vi "EncoderLimitsTurret.vi"(8 "Encoder Minimum Position":dbl, 9 "Encoder Maximum Position":dbl, 10 "Encoder Position":dbl, 11 "Output":dbl) -> (3 "Output":dbl)   [LabVIEW 2020]
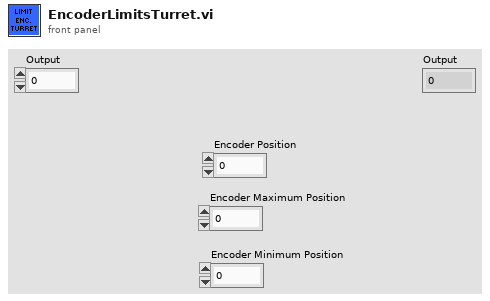
[diagram p1: front panel]
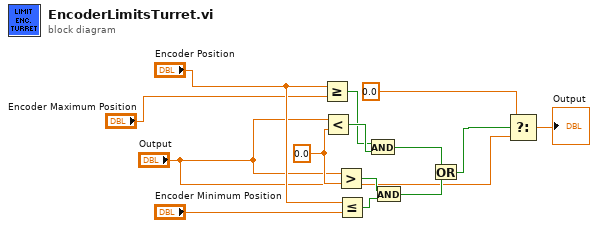
[diagram p0: block diagram]
diagram:
  w11 = 0.0 ("y")
  n1 = Greater Or Equal?(x="Encoder Position", y="Encoder Maximum Position") -> (x >= y?=w12:bool)
  n2 = Less?(x="Output", y=w11) -> (x < y?=w13:bool)
  n3 = Greater?(x="Output", y=w11) -> (0:w10:bool)
  n4 = Less Or Equal?(x="Encoder Position", y="Encoder Minimum Position") -> (x <= y?=w3:bool)
  n5 = And(x=w12, y=w13) -> (x .and. y?=w9:bool)
  n6 = And(x=w10, y=w3) -> (x .and. y?=w8:bool)
  n7 = Or(x=w9, y=w8) -> (x .or. y?=w7:bool)
  n8 = Select(t=0.0, s=w7, f="Output") -> (s? t:f=→"Output":dbl)
